vi "RunMeas.vi"(8 "error in (no error)":errorcluster, 11 "NHRDCPower in":refnum<class "NHRDCPower.lvclass">) -> (0 "error out":errorcluster, 2 "variant":variant, 3 "NHRDCPower out":refnum<class "NHRDCPower.lvclass">)   [LabVIEW 2018, in "AcPwrPlugins.lvlib" / "NHRDCPower.lvclass"]
doc: "This VI initiates and takes measurements from the instrument(s)."
uses:
  NHRDCPower.lvclass
  AcPwrShared/clAcPwrAttributes.ctl
  <instrlib>/NHRDCPowerModule/NHRDCPowerModule/NHRDCPowerModule.lvlib
  AcPwrShared/AcPwrShared.lvlib
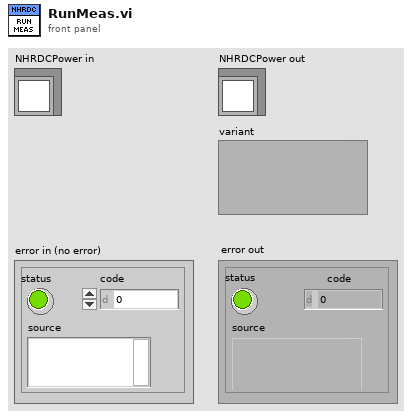
[diagram p1: front panel]
types:
  T1 = typedef "AcPwrPlugins.lvlib/NHRDCPower.lvclass/Measurements.ctl" = cluster{"Handle":string, "Name":string, "Enabled":bool, "Measurement Value":sgl, "Measurement Type":enum16{"Power", "Current", "Voltage"}}[]
  T2 = typedef "AcPwrShared.lvlib/clAcPwrAttributes.ctl" = cluster{"ProtectionStatusString":string, "Handle_MeasurementType":string, "Status Byte Register":cluster{"Busy":bool, "Remote Mode":bool, "Error in Queue":bool, "QUES=Questionable Status Summary":bool, "MAV = Message Available":bool, "ESB = Event Status Byte Summary":bool, "RQS = Request for Service":bool, "OPER = Operation Event Summary":bool}}
  T3 = cluster{"MeasName":string, "Variant":variant, "xml string":string}
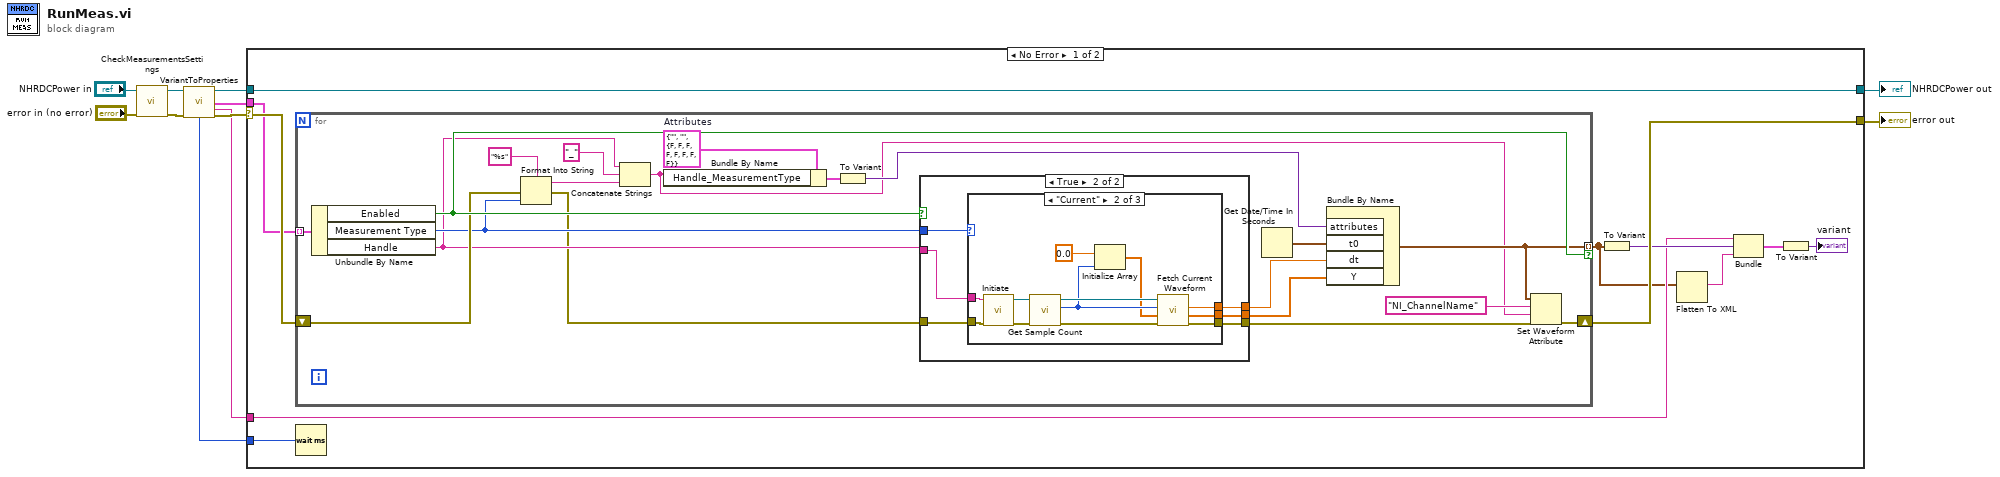
[diagram p0: block diagram]
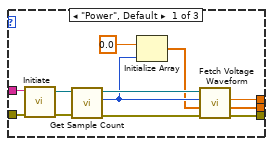
[diagram p3: hidden frame]
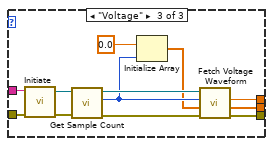
[diagram p4: hidden frame]
diagram:
  n1 = call-dynamic "CheckMeasurementsSettings.vi"("error in (no error)"="error in (no error)", "NHRDCPower in"="NHRDCPower in") -> ("error out"=w7:errorcluster, "NHRDCPower out"=w6:refnum<class "NHRDCPower.lvclass">)  [unwired: 8 in]
  n2 = call "VariantToProperties.vi"("NHRDCPower in"=w6, "error in (no error)"=w7) -> ("NHRDCPower out"=w4:refnum<class "NHRDCPower.lvclass">, "Meas"=w1:T1, "MeasName"=w3:string, "Measurement Refresh Time (ms)"=w2:u32, "error out"=w5:errorcluster)  [unwired: 7 in, 2 out]
  n3 = case shown="No Error" w5 {
    selector: w5 -> [w21 w86]
    tunnel: [w17 w86] -> w11
    tunnel: [w22 w87] -> w10
    tunnel: w4 -> [w22 w87]
    tunnel: w3 -> [w14 _]
    tunnel: w2 -> [w20 _]
    tunnel: w1 -> [w19 _]
    frame No Error {
      n4 = for {
        tunnel: w19 -> [w42] mode=indexing
        shift-right: [w26] -> w17
        shift-left: w21 -> [w32]
        tunnel: [w24] -> w12 mode=indexing if=w41
        w37 = T2 {"ProtectionStatusString"="", "Handle_MeasurementType"="", "Status Byte Register"={"Busy"=FALSE, "Remote Mode"=FALSE, "Error in Queue"=FALSE, "QUES=Questionable Status Summary"=FALSE, "MAV = Message Available"=FALSE, "ESB = Event Status Byte Summary"=FALSE, "RQS = Request for Service"=FALSE, "OPER = Operation Event Summary"=FALSE}}  # Attributes
        n5 = Unbundle By Name(w42) -> ("Enabled"=w41:bool, "Measurement Type"=w31:enum16{"Power", "Current", "Voltage"}, "Handle"=w30:string)
        n6 = Format Into String(format string="%s", error in=w32, w31) -> (resulting string=w33:string, error out=w28:errorcluster)  [unwired: 1 in]
        n7 = Concatenate Strings(w30, "_", w33) -> (w23:string)
        n8 = Bundle By Name(cluster=w37, "Handle_MeasurementType"=w23) -> (w36:T2)
        n9 = To Variant(anything=w36) -> (Variant=w29:variant)
        n10 = case shown="True" w41 {
          tunnel: w31 -> [_ w49]
          tunnel: w30 -> [_ w48]
          tunnel: w28 -> [w43 w47]
          tunnel: [w43 w46] -> w25
          tunnel: [_ w45] -> w39
          tunnel: [_ w44] -> w38
          frame False {
          }
          frame True {
            n11 = case shown="\"Current\"" w49 {
              tunnel: [w54 w66 w78] -> w46
              tunnel: [w53 w65 w77] -> w45
              tunnel: [w52 w64 w76] -> w44
              tunnel: w48 -> [w50 w63 w75]
              tunnel: w47 -> [w51 w62 w74]
              frame "Power", Default {
                n12 = call <instrlib>:"Initiate.vi"("error in (no error)"=w51, "instrument handle"=w50) -> ("error out"=w58:errorcluster, "instrument handle out"=w59:refnum<visa-resource-name>)  [unwired: 8 in]
                n13 = call <instrlib>:"Get Sample Count.vi"("error in (no error)"=w58, "instrument handle"=w59) -> ("error out"=w60:errorcluster, "sample count"=w57:i32, "instrument handle out"=w61:refnum<visa-resource-name>)  [unwired: 7 in]
                n14 = Initialize Array(sgl 0.0 ("Numeric"), w57) -> (w56:sgl[])
                n15 = call <instrlib>:"Fetch Voltage Waveform.vi"("error in (no error)"=w60, "voltage buffer"=w56, "voltage buffer size"=w57, "instrument handle"=w61) -> ("error out"=w54:errorcluster, "voltage"=w53:sgl[], "X increment"=w52:sgl)  [unwired: 3 in, 2 out]
              }
              frame "Current" {
                n16 = call <instrlib>:"Initiate.vi"("error in (no error)"=w62, "instrument handle"=w63) -> ("error out"=w70:errorcluster, "instrument handle out"=w71:refnum<visa-resource-name>)  [unwired: 8 in]
                n17 = call <instrlib>:"Get Sample Count.vi"("error in (no error)"=w70, "instrument handle"=w71) -> ("error out"=w72:errorcluster, "sample count"=w69:i32, "instrument handle out"=w73:refnum<visa-resource-name>)  [unwired: 7 in]
                n18 = Initialize Array(sgl 0.0 ("Numeric"), w69) -> (w68:sgl[])
                n19 = call <instrlib>:"Fetch Current Waveform.vi"("error in (no error)"=w72, "current buffer"=w68, "current buffer size"=w69, "instrument handle"=w73) -> ("error out"=w66:errorcluster, "current"=w65:sgl[], "X increment"=w64:sgl)  [unwired: 3 in, 2 out]
              }
              frame "Voltage" {
                n20 = call <instrlib>:"Initiate.vi"("error in (no error)"=w74, "instrument handle"=w75) -> ("error out"=w82:errorcluster, "instrument handle out"=w83:refnum<visa-resource-name>)  [unwired: 8 in]
                n21 = call <instrlib>:"Get Sample Count.vi"("error in (no error)"=w82, "instrument handle"=w83) -> ("error out"=w84:errorcluster, "sample count"=w81:i32, "instrument handle out"=w85:refnum<visa-resource-name>)  [unwired: 7 in]
                n22 = Initialize Array(sgl 0.0 ("Numeric"), w81) -> (w80:sgl[])
                n23 = call <instrlib>:"Fetch Voltage Waveform.vi"("error in (no error)"=w84, "voltage buffer"=w80, "voltage buffer size"=w81, "instrument handle"=w85) -> ("error out"=w78:errorcluster, "voltage"=w77:sgl[], "X increment"=w76:sgl)  [unwired: 3 in, 2 out]
              }
            }
          }
        }
        n24 = Get Date/Time In Seconds() -> (seconds since 1Jan1904=w40:timestamp)
        n25 = Bundle By Name("attributes"=w29, "t0"=w40, "dt"=w38, "Y"=w39) -> (w24:waveform(sgl))  [unwired: 1 in]
        n26 = Set Waveform Attribute(4:w25, 5:w23, 6:"NI_ChannelName" ("name"), 7:w24) -> (0:w26:errorcluster)  [unwired: 2 out]
      }
      n27 = Wait (ms)(milliseconds to wait=w20) -> ()  [unwired: 1 out]
      n28 = To Variant(anything=w12) -> (Variant=w15:variant)
      n29 = Flatten To XML(anything=w12) -> (xml string=w13:string)
      n30 = Bundle("MeasName"=w14, "Variant"=w15, "xml string"=w13) -> (w16:T3)  [unwired: 1 in]
      n31 = To Variant(anything=w16) -> (Variant=→"variant":variant)
    }
    frame Error {
    }
  }
  "NHRDCPower out" <- w10
  "error out" <- w11
